vi "设置电压并读取.vi"(7 "布尔":bool, 8 "error out":errorcluster, 9 "V2设置值":i32, 10 "V1设置值":i32, 11 "VISA resource name out":refnum<visa-resource-name>) -> (0 "V2当前电压":dbl format="%_6g", 1 "V1当前电压":dbl format="%_6g", 2 "V2_Digital":string, 3 "V1_Digital":string)   [LabVIEW 2018]
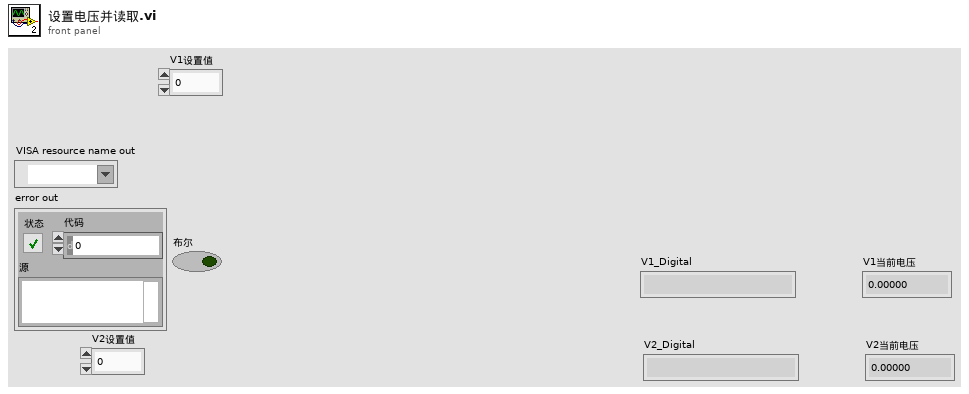
[diagram p1: front panel]
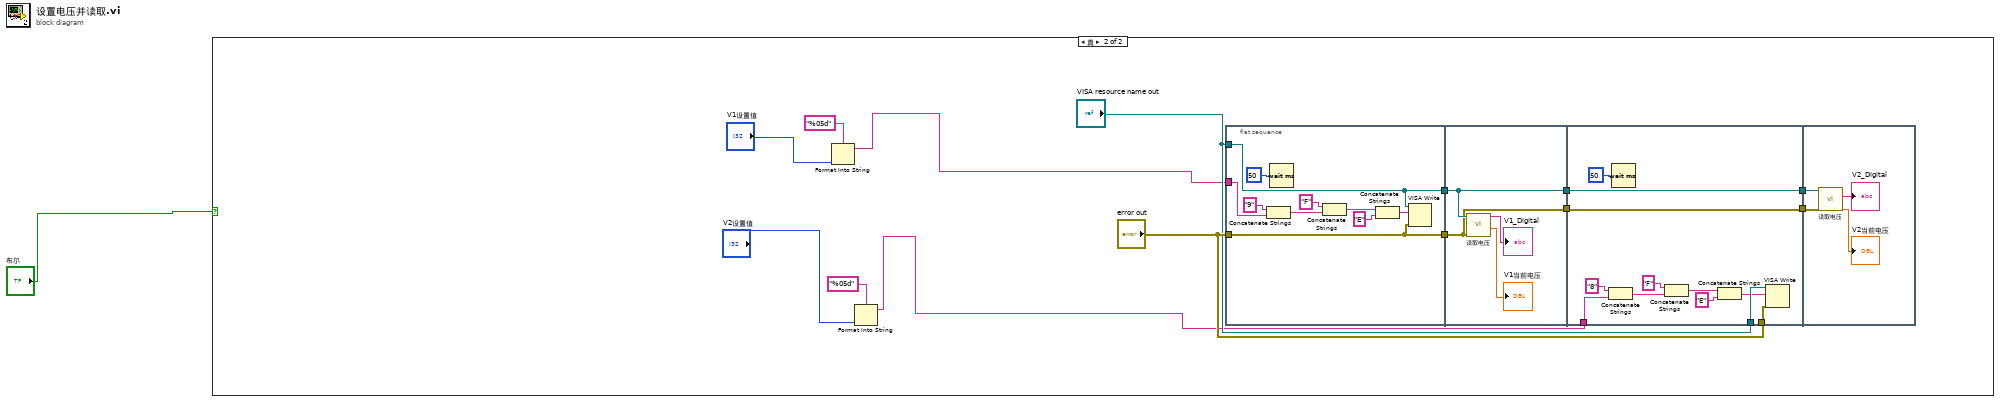
[diagram p0: block diagram]
diagram:
  n1 = case shown="真" "布尔" {
    frame False {
    }
    frame True {
      n2 = Format Into String(format string="%05d" ("格式字符串"), "V1设置值") -> (resulting string=w5:string)  [unwired: 2 in, 1 out]
      n3 = Format Into String(format string="%05d" ("格式字符串"), "V2设置值") -> (resulting string=w2:string)  [unwired: 2 in, 1 out]
      n4 = flat-sequence {
        tunnel: "VISA resource name out" -> [w17]
        tunnel: "error out" -> [w16]
        tunnel: w5 -> [w18]
        tunnel: [w17] -> w15
        tunnel: [w16] -> w14
        tunnel: w15 -> [w27]
        tunnel: w14 -> [w26]
        tunnel: [w27] -> w13
        tunnel: [w26] -> w12
        tunnel: "error out" -> [w40]
        tunnel: "VISA resource name out" -> [w39]
        tunnel: w2 -> [w32]
        tunnel: [w31] -> w11
        tunnel: w13 -> [w31]
        tunnel: w12 -> [w30]
        tunnel: [w30] -> w10
        tunnel: w11 -> [w45]
        tunnel: w10 -> [w44]
        frame #0 {
          n5 = Concatenate Strings("9", w18) -> (w22:string)
          n6 = Wait (ms)(milliseconds to wait=50) -> ()  [unwired: 1 out]
          n7 = Concatenate Strings("F", w22) -> (w20:string)
          n8 = Concatenate Strings(w20, "E") -> (w19:string)
          n9 = VISA Write(VISA resource name=w17, write buffer=w19, error in (no error)=w16) -> ()  [unwired: 3 out]
        }
        frame #1 {
          n10 = call "读取电压.vi"("错误输入（无错误）"=w26, "VISA资源名称"=w27) -> ("V1当前电压"=→"V1当前电压":dbl, "V1_Digital"=→"V1_Digital":string)  [unwired: 6 in, 2 out]
        }
        frame #2 {
          n11 = Concatenate Strings("8", w32) -> (w35:string)
          n12 = Wait (ms)(milliseconds to wait=50) -> ()  [unwired: 1 out]
          n13 = Concatenate Strings("F", w35) -> (w36:string)
          n14 = Concatenate Strings(w36, "E") -> (w33:string)
          n15 = VISA Write(VISA resource name=w39, write buffer=w33, error in (no error)=w40) -> ()  [unwired: 3 out]
        }
        frame #3 {
          n16 = call "读取电压.vi"("错误输入（无错误）"=w44, "VISA资源名称"=w45) -> ("V2当前电压"=→"V2当前电压":dbl, "V2_Digital"=→"V2_Digital":string)  [unwired: 6 in, 2 out]
        }
      }
    }
  }
